vi "FPGA_PPG_getting_started.vi"() -> ()   [LabVIEW 2014, in "NI-FPGA_PPG_Driver.lvlib"]
doc: "Provides a simple test to check the communication with the FPGA card by querying the firmware revision.\n\nDietrich Beck, GSI Helmholtzzentrum fuer Schwerionenforschung, Germany"
uses:
  NI-FPGA_PPG_Driver.lvlib
panel:
  out "clockRate [ticks/us]":i32
  out "revision":string
  in  "resource_in":refnum<visa-resource-name>
  out "error out":errorcluster
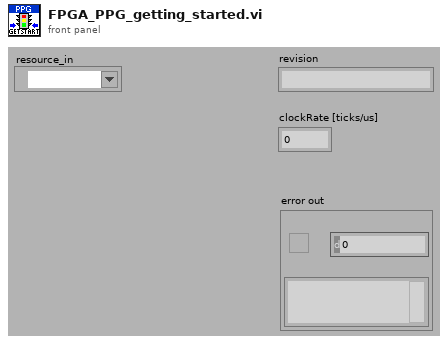
[diagram p1: front panel]
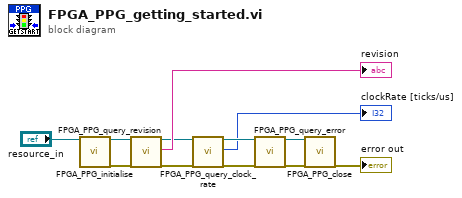
[diagram p0: block diagram]
diagram:
  n1 = call "FPGA_PPG_initialise.vi"("resource_in"="resource_in") -> ("resource_out"=w12:refnum<visa-resource-name>, "error out"=w1:errorcluster)  [unwired: 16 in, 1 out]
  n2 = call "FPGA_PPG_query_revision.vi"("resource_in"=w12, "error in (no error)"=w1) -> ("resource_out"=w3:refnum<visa-resource-name>, "revision"=→"revision":string, "error out"=w6:errorcluster)  [unwired: 15 in]
  n3 = call "FPGA_PPG_query_clock_rate.vi"("resource_in"=w3, "error in (no error)"=w6) -> ("resource_out"=w4:refnum<visa-resource-name>, "clockRate [ticks/us]"=→"clockRate [ticks/us]":i32, "error out"=w5:errorcluster)  [unwired: 15 in]
  n4 = call "FPGA_PPG_query_error.vi"("resource_in"=w4, "error in (no error)"=w5) -> ("resource_out"=w8:refnum<visa-resource-name>, "error out"=w9:errorcluster)  [unwired: 16 in]
  n5 = call "FPGA_PPG_close.vi"("resource_in"=w8, "error in (no error)"=w9) -> ("error out"=→"error out":errorcluster)  [unwired: 17 in]
